vi "G to e2h (2D).vi"(8 "error in (no error)":errorcluster, 10 "e^2/h?":bool, 11 "Array in":dbl[][](array[numeric])) -> (0 "error out":errorcluster, 3 "Array out":dbl[][](array[numeric]))   [LabVIEW 2016, in "Retrieve and Visualize.lvclass"]
uses:
  Retrieve and Visualize.lvclass
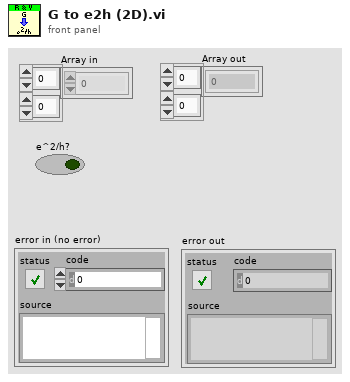
[diagram p1: front panel]
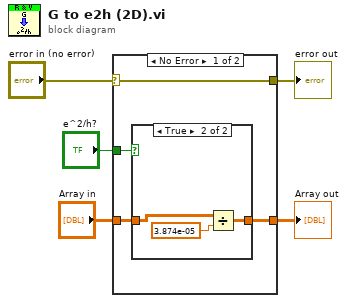
[diagram p0: block diagram]
diagram:
  n1 = case shown="No Error" "error in (no error)" {
    selector: "error in (no error)" -> [w6 w15]
    tunnel: [w9 w14] -> w5
    tunnel: "Array in" -> [w8 w14]
    tunnel: "e^2/h?" -> [w7 _]
    tunnel: [w6 w15] -> w1
    frame No Error {
      n2 = case shown="True" w7 {
        tunnel: w8 -> [w10 w13]
        tunnel: [w10 w12] -> w9
        frame False {
        }
        frame True {
          n3 = Divide(x=w13, y=3.874e-05) -> (x/y=w12:dbl[][])
        }
      }
    }
    frame Error {
    }
  }
  "Array out" <- w5
  "error out" <- w1
